vi "OP600ZP_Assembly.vi"(8 "DCIR_MESURES":cluster{dbl, dbl, dbl, dbl, dbl, dbl, dbl, dbl}) -> (1 "Out":string, 3 "PASS/FAIL":bool)   [LabVIEW 2020]
uses:
  OP600ZP_VGConf.vi
  VG/PackType.vi
  VG/IS30%.vi
  VG/DCIR@1C.vi
  VG/Ubatt.vi
panel:
  out "errout":errorcluster caption="error out"
  in  "errin":errorcluster caption="error out"
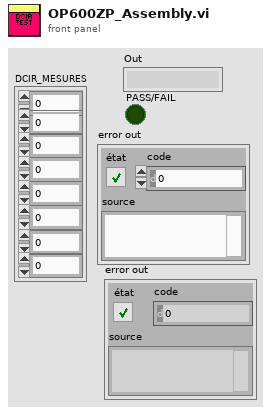
[diagram p1: front panel]
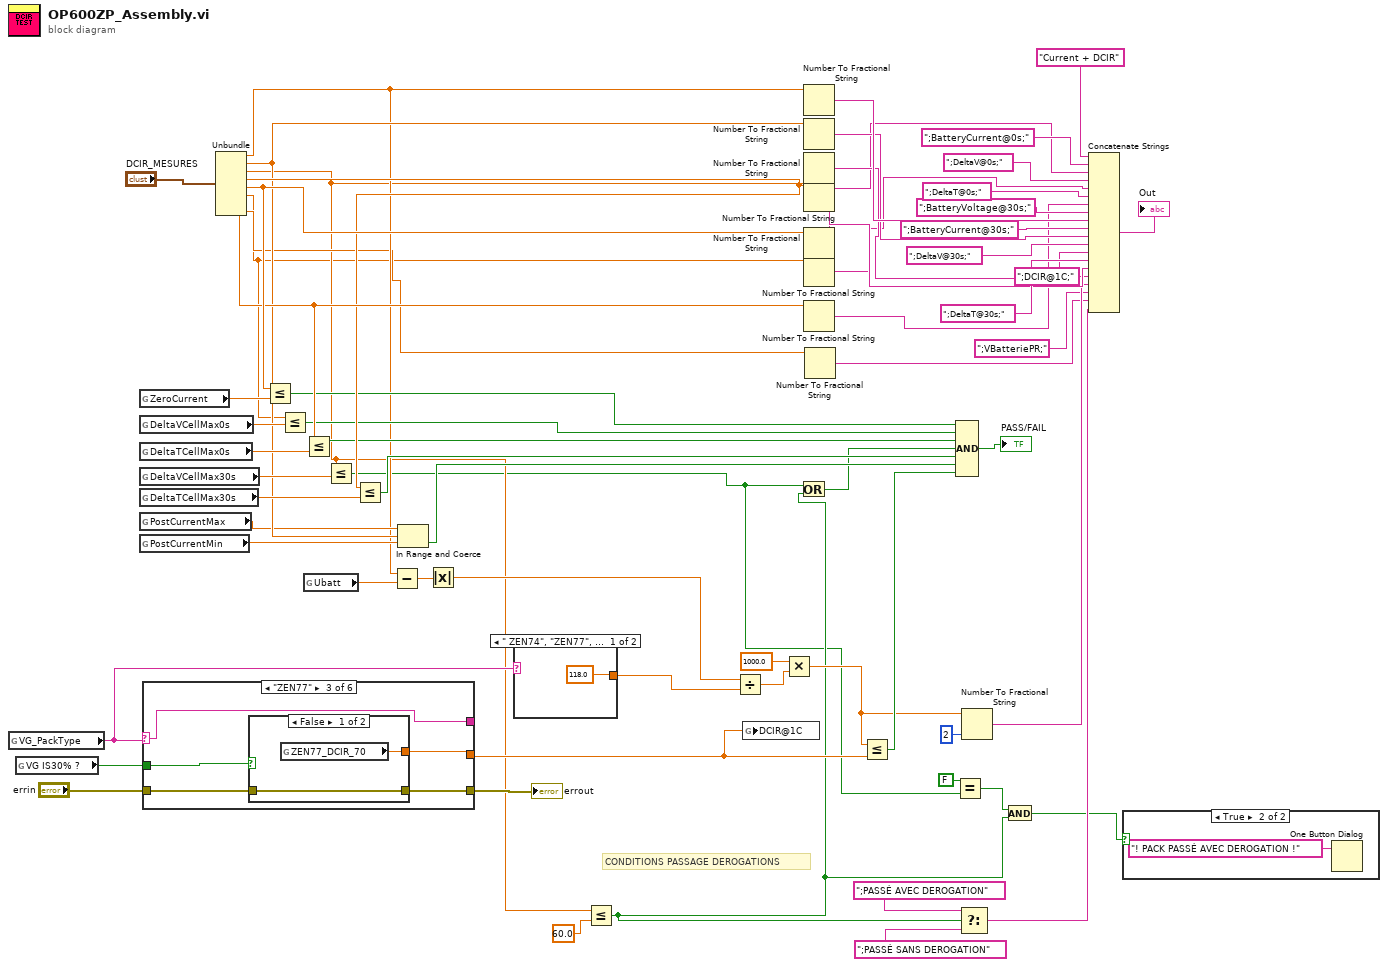
[diagram p0: block diagram]
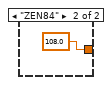
[diagram p3: hidden frame]
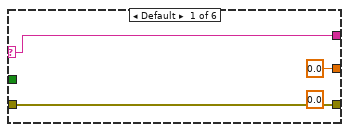
[diagram p4: hidden frame]
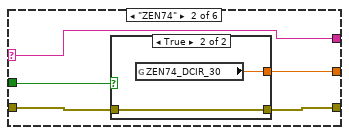
[diagram p5: hidden frame]
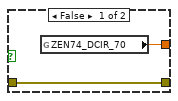
[diagram p6: hidden frame]
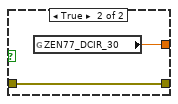
[diagram p7: hidden frame]
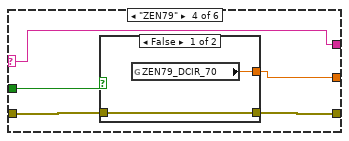
[diagram p8: hidden frame]
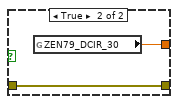
[diagram p9: hidden frame]
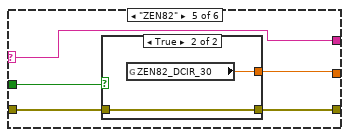
[diagram p10: hidden frame]
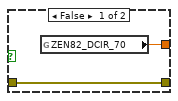
[diagram p11: hidden frame]
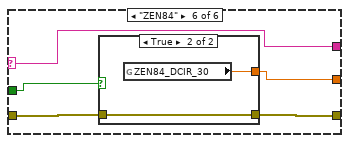
[diagram p12: hidden frame]
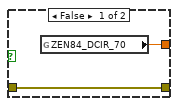
[diagram p13: hidden frame]
diagram:
  # "CONDITIONS PASSAGE DEROGATIONS"
  n1 = global read "PackType.vi" "VG_PackType"() -> (w26:string)
  n2 = global read "IS30%.vi" "VG IS30% ?"() -> (w32:bool)
  n3 = global read "OP600ZP_VGConf.vi" "ZeroCurrent"() -> (w65:dbl)
  n4 = global read "OP600ZP_VGConf.vi" "DeltaVCellMax0s"() -> (w53:dbl)
  n5 = global read "OP600ZP_VGConf.vi" "DeltaTCellMax0s"() -> (w52:dbl)
  n6 = global read "OP600ZP_VGConf.vi" "DeltaVCellMax30s"() -> (w50:dbl)
  n7 = global read "OP600ZP_VGConf.vi" "DeltaTCellMax30s"() -> (w49:dbl)
  n8 = global read "OP600ZP_VGConf.vi" "PostCurrentMax"() -> (w46:dbl)
  n9 = global read "OP600ZP_VGConf.vi" "PostCurrentMin"() -> (w45:dbl)
  n10 = case shown="\"ZEN77\"" w26 {
    selector: w26 -> [w69 w72 w81 w90 w99 w108]
    tunnel: [0.0 ("ZEN84UbattMax30") w74 w83 w92 w101 w110] -> w21
    tunnel: w32 -> [_ w73 w82 w91 w100 w109]
    tunnel: [w69 w72 w81 w90 w99 w108] -> _
    tunnel: "errin" -> [w68 w71 w80 w89 w98 w107]
    tunnel: [w68 w70 w79 w88 w97 w106] -> w30
    frame Default {
      (unwired) 0.0 ("ZEN84UbattMin30")
    }
    frame "ZEN74" {
      n11 = case shown="True" w73 {
        tunnel: [w76 w78] -> w74
        tunnel: [w75 w77] -> w70
        tunnel: w71 -> [w75 w77]
        frame False {
          n12 = global read "OP600ZP_VGConf.vi" "ZEN74_DCIR_70"() -> (w76:dbl)
        }
        frame True {
          n13 = global read "OP600ZP_VGConf.vi" "ZEN74_DCIR_30"() -> (w78:dbl)
        }
      }
    }
    frame "ZEN77" {
      n14 = case shown="False" w82 {
        tunnel: [w85 w87] -> w83
        tunnel: w80 -> [w84 w86]
        tunnel: [w84 w86] -> w79
        frame False {
          n15 = global read "OP600ZP_VGConf.vi" "ZEN77_DCIR_70"() -> (w85:dbl)
        }
        frame True {
          n16 = global read "OP600ZP_VGConf.vi" "ZEN77_DCIR_30"() -> (w87:dbl)
        }
      }
    }
    frame "ZEN79" {
      n17 = case shown="False" w91 {
        tunnel: [w94 w96] -> w92
        tunnel: w89 -> [w93 w95]
        tunnel: [w93 w95] -> w88
        frame False {
          n18 = global read "OP600ZP_VGConf.vi" "ZEN79_DCIR_70"() -> (w94:dbl)
        }
        frame True {
          n19 = global read "OP600ZP_VGConf.vi" "ZEN79_DCIR_30"() -> (w96:dbl)
        }
      }
    }
    frame "ZEN82" {
      n20 = case shown="True" w100 {
        tunnel: [w103 w105] -> w101
        tunnel: w98 -> [w102 w104]
        tunnel: [w102 w104] -> w97
        frame False {
          n21 = global read "OP600ZP_VGConf.vi" "ZEN82_DCIR_70"() -> (w103:dbl)
        }
        frame True {
          n22 = global read "OP600ZP_VGConf.vi" "ZEN82_DCIR_30"() -> (w105:dbl)
        }
      }
    }
    frame "ZEN84" {
      n23 = case shown="True" w109 {
        tunnel: [w112 w114] -> w110
        tunnel: w107 -> [w111 w113]
        tunnel: [w111 w113] -> w106
        frame False {
          n24 = global read "OP600ZP_VGConf.vi" "ZEN84_DCIR_70"() -> (w112:dbl)
        }
        frame True {
          n25 = global read "OP600ZP_VGConf.vi" "ZEN84_DCIR_30"() -> (w114:dbl)
        }
      }
    }
  }
  "errout" <- w30
  n26 = Unbundle("DCIR_MESURES") -> (w29:dbl, w47:dbl, w10:dbl, w48:dbl, w55:dbl, w9:dbl, w51:dbl, w15:dbl)
  n27 = Less Or Equal?(x=w55, y=w65) -> (x <= y?=w44:bool)
  n28 = Less Or Equal?(x=w9, y=w53) -> (x <= y?=w43:bool)
  n29 = Less Or Equal?(x=w51, y=w52) -> (x <= y?=w42:bool)
  n30 = global read "Ubatt.vi" "Ubatt"() -> (w28:dbl)
  n31 = Less Or Equal?(x=w10, y=w50) -> (x <= y?=w3:bool)
  n32 = Less Or Equal?(x=w48, y=w49) -> (x <= y?=w41:bool)
  n33 = Subtract(x=w29, y=w28) -> (x-y=w27:dbl)
  n34 = In Range and Coerce(upper limit=w46, x=w47, lower limit=w45) -> (In Range?=w40:bool)  [unwired: 1 out]
  n35 = Absolute Value(x=w27) -> (abs(x)=w25:dbl)
  n36 = case shown="\" ZEN74\", \"ZEN77\", \"ZEN79\", \"ZEN82\", Default" w26 {
    tunnel: [118.0 108.0] -> w19
    frame " ZEN74", "ZEN77", "ZEN79", "ZEN82", Default {
    }
    frame "ZEN84" {
    }
  }
  n37 = Less Or Equal?(x=w10, y=60.0) -> (x <= y?=w11:bool)
  n38 = Divide(x=w25, y=w19) -> (x/y=w17:dbl)
  n39 = global write "DCIR@1C.vi" "DCIR@1C"(w21) -> ()
  n40 = Multiply(x=1000.0, y=w17) -> (x*y=w16:dbl)
  n41 = Or(x=w3, y=w11) -> (x .or. y?=w5:bool)
  n42 = Number To Fractional String(number=w29) -> (F-format string=w39:string)  [unwired: 3 in]
  n43 = Number To Fractional String(number=w47) -> (F-format string=w38:string)  [unwired: 3 in]
  n44 = Number To Fractional String(number=w10) -> (F-format string=w37:string)  [unwired: 3 in]
  n45 = Number To Fractional String(number=w48) -> (F-format string=w36:string)  [unwired: 3 in]
  n46 = Number To Fractional String(number=w55) -> (F-format string=w33:string)  [unwired: 3 in]
  n47 = Number To Fractional String(number=w9) -> (F-format string=w35:string)  [unwired: 3 in]
  n48 = Number To Fractional String(number=w51) -> (F-format string=w34:string)  [unwired: 3 in]
  n49 = Number To Fractional String(number=w15) -> (F-format string=w13:string)  [unwired: 3 in]
  n50 = Less Or Equal?(x=w16, y=w21) -> (x <= y?=w20:bool)
  n51 = Equal?(x=FALSE, y=w3) -> (x = y?=w2:bool)
  n52 = Compound Arithmetic op=AND ("Opérateur arithmétique")(w44, w43, w42, w5, w41, w40, w20) -> (→"PASS/FAIL":bool)
  n53 = Select(t=";PASSÉ AVEC DEROGATION", s=w11, f=";PASSÉ SANS DEROGATION") -> (s? t:f=w6:string)
  n54 = Number To Fractional String(number=w16, precision (6)=i16 2 ("précision (6)")) -> (F-format string=w22:string)  [unwired: 2 in]
  n55 = And(x=w2, y=w11) -> (x .and. y?=w1:bool)
  n56 = Concatenate Strings("Current + DCIR" ("élément"), ";BatteryCurrent@0s;" ("élément"), w33, ";DeltaV@0s;" ("élément"), w35, ";DeltaT@0s;" ("élément"), w34, ";BatteryVoltage@30s;" ("élément"), w39, ";BatteryCurrent@30s;" ("élément"), w38, ";DeltaV@30s;" ("élément"), w37, ";DeltaT@30s;" ("élément"), w36, ";DCIR@1C;" ("chaîne"), w22, ";VBatteriePR;" ("chaîne"), w13, w6) -> (→"Out":string)
  n57 = case shown="True" w1 {
    frame False {
    }
    frame True {
      n58 = One Button Dialog(message="! PACK PASSÉ AVEC DEROGATION !") -> ()  [unwired: 1 in, 1 out]
    }
  }
